vi "getConfig.vi"(6 "Delay between send and receive [ms]":i32=100, 8 "error in (no error)":errorcluster, 11 "CCD in":refnum<class "CCD.lvclass">) -> (0 "error out":errorcluster, 1 "config data":T1={"centerWavelength"=0.0, "chipHSpacing"=0.0, "chipHeight"=0.0, "chipName"="$.configuration", "chipSerialNumber"="$.configuration", "chipVSpacing"=0.0, "chipWidth"=0.0, "deviceType"="$.configuration", "fitParameters"=[], "gains"=[], "hardwareAvgAvailable"=FALSE, "lineScan"=FALSE, "productId"="$.configuration", "serialNumber"="", "signals"=[], "speeds"=[], "supportedFeatures"={"cf_3PositionSlit"=FALSE, "cf_CMOSOffsetCorrection"=FALSE, "cf_Cleaning"=FALSE, "cf_DSP"=FALSE, "cf_DSPBin2X"=FALSE, "cf_DelayAfterTrigger"=FALSE, "cf_Delays"=FALSE, "cf_EMCCD"=FALSE, "cf_EShutter"=FALSE, "cf_HDR"=FALSE, "cf_Image"=FALSE, "cf_MemorySlots"=FALSE, "cf_Metadata"=FALSE, "cf_MultipleExposeTimes"=FALSE, "cf_MultipleSensors"=FALSE, "cf_PulseSummation"=FALSE, "cf_ROIs"=FALSE, "cf_Signals"=FALSE, "cf_Spectra"=FALSE, "cf_TriggerQualifier"=FALSE, "cf_Triggers"=FALSE}, "triggers"=[], "version"=""}, 2 "config-JSON string":string, 3 "CCD out":refnum<class "CCD.lvclass">)   [LabVIEW 2023, in "CCD.lvclass"]
doc: "Returns the CCD device configuration.\n\nresults description\nconfiguration JSON. CCD device configuration.\n\nxample response:\n\n{\n \"command\": \"ccd_getConfig\",\n \"errors\": [],\n \"id\": 1234,\n \"results\": {\n \"configuration\": {\n \"chipHSpacing\": \"140\",\n \"chipHeight\": \"70\",\n \"chipName\": \"S10420\",\n \"chipSerialNumber\": \"FAH23 098\",\n \"chipVSpacing\": \"140\",\n \"chipWidth\": \"2048\",\n \"deviceType\": \"HORIBA Scientific Syncerity\",\n \"fitParameters\": [\n 0,\n 1,\n 0,\n 0,\n 0\n ],\n \"gains\": [\n {\n \"info\": \"Best Dynamic Range\",\n \"token\": 1\n },\n {\n \"info\": \"High Sensitivity\",\n \"token\": 2\n },\n {\n \"info\": \"High Light\",\n \"token\": 0\n }\n ],\n \"hardwareAvgAvailable\": false,\n \"lineScan\": false,\n \"parallelSpeeds\": [\n {\n \"info\": \"9.6 µSec\",\n \"token\": 1\n },\n {\n \"info\": \"4.9 µSec\",\n \"token\": 2\n },\n {\n \"info\": \"19 µSec\",\n \"token\": 0\n }\n ],\n \"productId\": \"13\",\n \"serialNumber\": \"Camera SN: 5128\",\n \"signals\": [\n {\n \"events\": [\n {\n \"name\": \"Ready For Trigger\",\n \"token\": 1,\n \"types\": [\n {\n \"name\": \"TTL Active Low\",\n \"token\": 1\n },\n {\n \"name\": \"TTL Active High\",\n \"token\": 0\n }\n ]\n },\n {\n \"name\": \"Not Readout\",\n \"token\": 2,\n \"types\": [\n {\n \"name\": \"TTL Active Low\",\n \"token\": 1\n },\n {\n \"name\": \"TTL Active High\",\n \"token\": 0\n }\n ]\n },\n {\n \"name\": \"Shutter Open\",\n \"token\": 3,\n \"types\": [\n {\n \"name\": \"TTL Active Low\",\n \"token\": 1\n },\n {\n \"name\": \"TTL Active High\",\n \"token\": 0\n }\n ]\n },\n {\n \"name\": \"Start Experiment\",\n \"token\": 0,\n \"types\": [\n {\n \"name\": \"TTL Active Low\",\n \"token\": 1\n },\n {\n \"name\": \"TTL Active High\",\n \"token\": 0\n }\n ]\n }\n ],\n \"name\": \"Signal Output\",\n \"token\": 0\n }\n ],\n \"speeds\": [\n {\n \"info\": \"500 kHz \",\n \"token\": 1\n },\n {\n \"info\": \"500 kHz Ultra\",\n \"token\": 2\n },\n {\n \"info\": \"500 kHz Wrap\",\n \"token\": 127\n },\n {\n \"info\": \" 45 kHz \",\n \"token\": 0\n }\n ],\n \"supportedFeatures\": {\n \"cf_3PositionSlit\": false,\n \"cf_CMOSOffsetCorrection\": false,\n \"cf_Cleaning\": true,\n \"cf_DSP\": false,\n \"cf_DSPBin2X\": false,\n \"cf_DelayAfterTrigger\": false,\n \"cf_Delays\": false,\n \"cf_EMCCD\": false,\n \"cf_EShutter\": false,\n \"cf_HDR\": false,\n \"cf_Image\": true,\n \"cf_MemorySlots\": true,\n \"cf_Metadata\": false,\n \"cf_MultipleExposeTimes\": false,\n \"cf_MultipleSensors\": false,\n \"cf_PulseSummation\": false,\n \"cf_ROIs\": true,\n \"cf_Signals\": true,\n \"cf_Spectra\": true,\n \"cf_TriggerQualifier\": false,\n \"cf_Triggers\": true\"\n },\n \"triggers\": [\n {\n \"events\": [\n {\n \"name\": \"Each - For Each Acq\",\n \"token\": 1,\n \"types\": [\n {\n \"name\": \"TTL Rising Edge\",\n \"token\": 1\n },\n {\n \"name\": \"TTL Falling Edge\",\n \"token\": 0\n }\n ]\n },\n {\n \"name\": \"Once - Start All\",\n \"token\": 0,\n \"types\": [\n {\n \"name\": \"TTL Rising Edge\",\n \"token\": 1\n },\n {\n \"name\": \"TTL Falling Edge\",\n \"token\": 0\n }\n ]\n }\n ],\n \"name\": \"Trigger Input\",\n \"token\": 0\n }\n ],\n \"version\": \"Syncerity Ver 1.002.9\"\n }\n }\n}"
uses:
  CCD.lvclass
  CCD.lvclass/CCD.ctl
  20f7d3bd-08ac-4524-9bed-df36c1da25a0.vi
  GenericDevice/GenericDevice.lvclass
  <vilib>/JDP Science/JSONtext/JSONtext.lvlib
  Gain.ctl
  Speed.ctl
  Type.ctl
  Event.ctl
  Signal.ctl
  Trigger.ctl
  SupportedFeatures.ctl
  GetConfig.ctl
panel:
  # "Connector Pane"
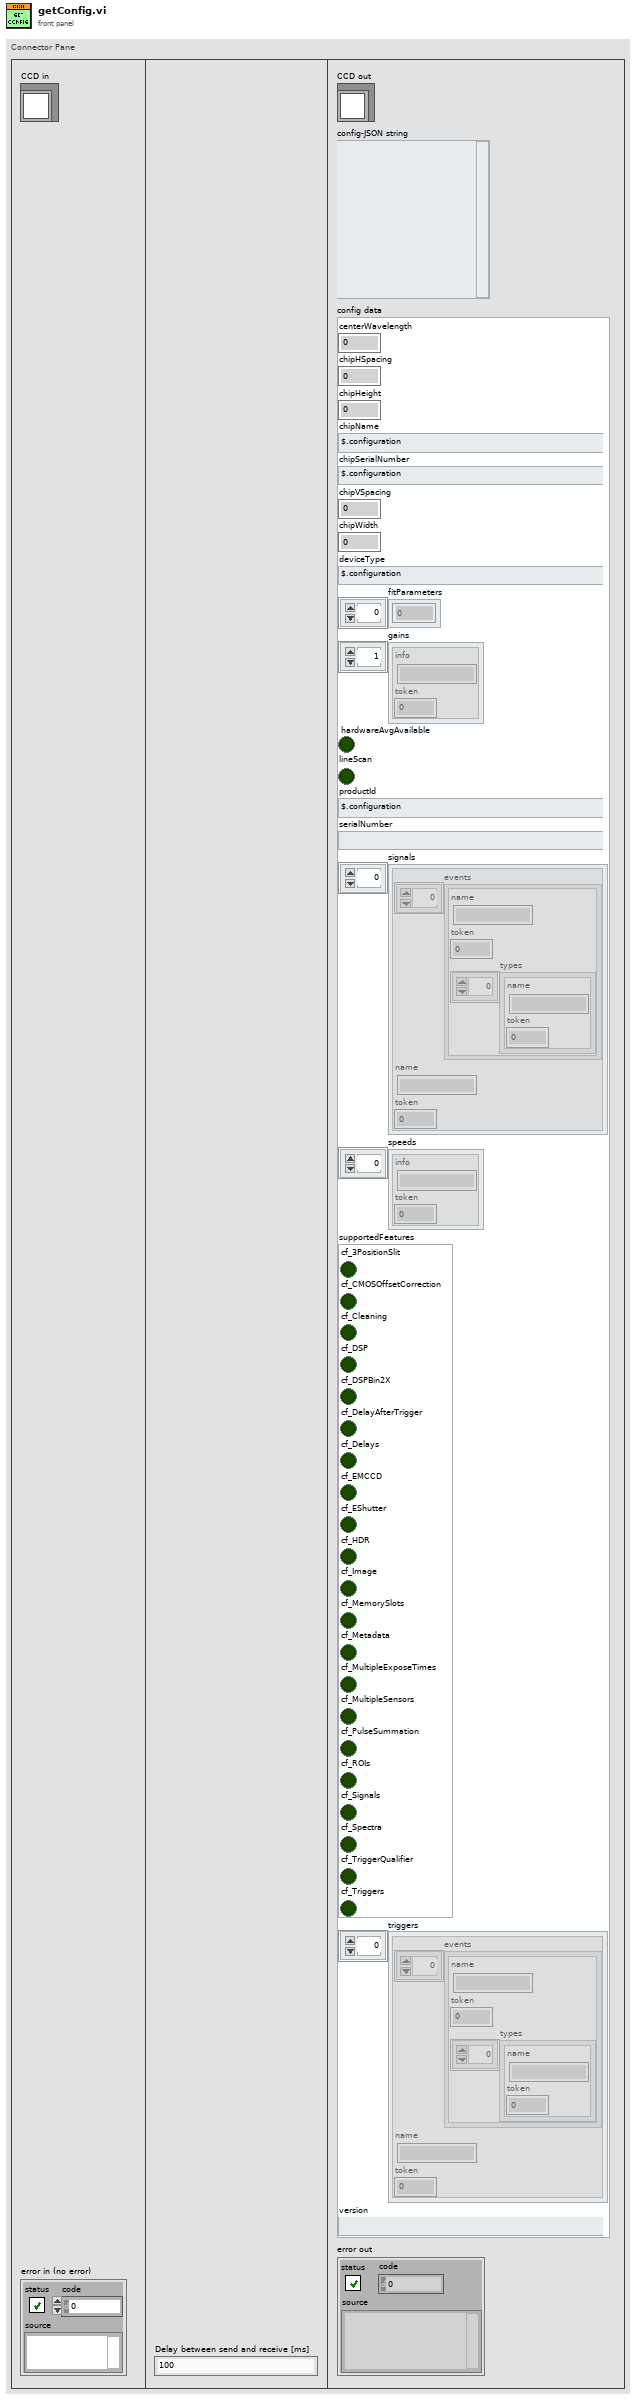
[diagram p1: front panel]
types:
  T1 = typedef "CCD.lvclass/GetConfig.ctl" = cluster{"centerWavelength":dbl, "chipHSpacing":dbl, "chipHeight":dbl, "chipName":string, "chipSerialNumber":string, "chipVSpacing":dbl, "chipWidth":dbl, "deviceType":string, "fitParameters":dbl[], "gains":T2[], "hardwareAvgAvailable":bool, "lineScan":bool, "productId":string, "serialNumber":string, "signals":T3[], "speeds":T6[], "supportedFeatures":T7, "triggers":T8[], "version":string}
  T2 = typedef "CCD.lvclass/Gain.ctl" = cluster{"info":string, "token":i32}
  T3 = typedef "CCD.lvclass/Signal.ctl" = cluster{"events":T4[], "name":string, "token":i32}
  T4 = typedef "CCD.lvclass/Event.ctl" = cluster{"name":string, "token":i32, "types":T5[]}
  T5 = typedef "CCD.lvclass/Type.ctl" = cluster{"name":string, "token":i32}
  T6 = typedef "CCD.lvclass/Speed.ctl" = cluster{"info":string, "token":i32}
  T7 = typedef "CCD.lvclass/SupportedFeatures.ctl" = cluster{"cf_3PositionSlit":bool, "cf_CMOSOffsetCorrection":bool, "cf_Cleaning":bool, "cf_DSP":bool, "cf_DSPBin2X":bool, "cf_DelayAfterTrigger":bool, "cf_Delays":bool, "cf_EMCCD":bool, "cf_EShutter":bool, "cf_HDR":bool, "cf_Image":bool, "cf_MemorySlots":bool, "cf_Metadata":bool, "cf_MultipleExposeTimes":bool, "cf_MultipleSensors":bool, "cf_PulseSummation":bool, "cf_ROIs":bool, "cf_Signals":bool, "cf_Spectra":bool, "cf_TriggerQualifier":bool, "cf_Triggers":bool}
  T8 = typedef "CCD.lvclass/Trigger.ctl" = cluster{"events":T4[], "name":string, "token":i32}
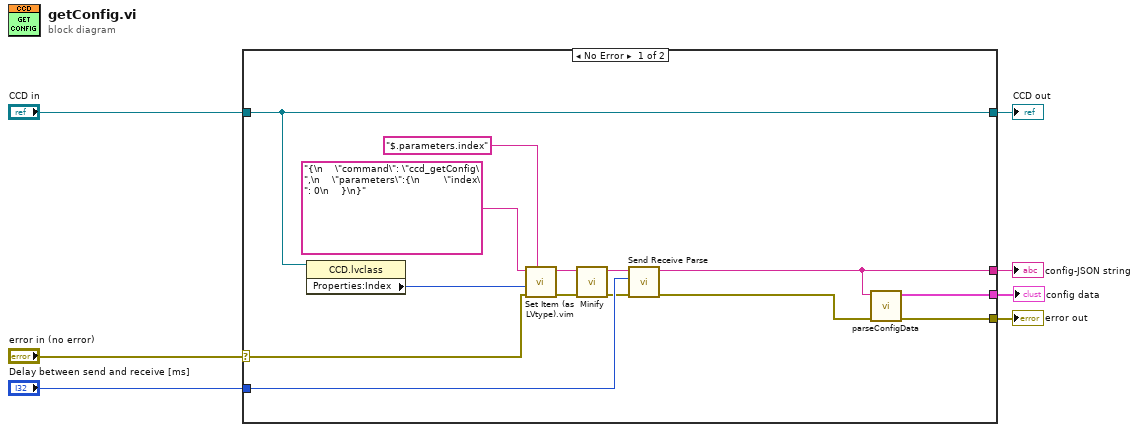
[diagram p0: block diagram]
diagram:
  n1 = case shown="No Error" "error in (no error)" {
    selector: "error in (no error)" -> [w17 w23]
    tunnel: [w12 w23] -> w6
    tunnel: [w19 w22] -> w4
    tunnel: "CCD in" -> [w19 w22]
    tunnel: [w14 _] -> w2
    tunnel: "Delay between send and receive [ms]" -> [w15 _]
    tunnel: [w11 _] -> w1
    frame No Error {
      n2 = property class="CCD.lvclass"(reference=w19) -> ("Properties:Index"=w18:i32)  [unwired: 1 in, 2 out]
      n3 = call "Set Item (as LVtype).vim"("$Path or Item Name"="$.parameters.index", "error in (no error)"=w17, "Anything"=w18, "JSON"="{\n    \"command\": \"ccd_getConfig\",\n    \"parameters\":{\n        \"index\": 0\n    }\n}") -> ("error out"=w16:errorcluster, "<JSON>"=w9:string)  [unwired: 4 in, 1 out]
      n4 = call <vilib>:"Minify.vi"("error in (no error)"=w16, "JSON"=w9) -> ("error out"=w10:errorcluster, "<JSON>"=w8:string)  [unwired: 7 in, 1 out]
      n5 = call "Send Receive Parse.vi"("error in"=w10, "Delay between send and receive [ms]"=w15, "<JSON>"=w8) -> ("error out"=w13:errorcluster, "results-JSON string"=w14:string)  [unwired: 6 in, 1 out]
      n6 = call "parseConfigData.vi"("error in (no error)"=w13, "results-JSON string"=w14) -> ("error out"=w12:errorcluster, "config data"=w11:T1)  [unwired: 6 in, 2 out]
    }
    frame Error {
    }
  }
  "error out" <- w6
  "CCD out" <- w4
  "config-JSON string" <- w2
  "config data" <- w1
